vi "PipBoy_ConvertImageToIcon.vi"(8 "error in (no error)":errorcluster, 10 "Image":T1) -> (0 "error out":errorcluster, 2 "Icon":u16[][](array[numeric]))   [LabVIEW 2014]
uses:
  <vilib>/picture/picture.llb/imagedata.ctl
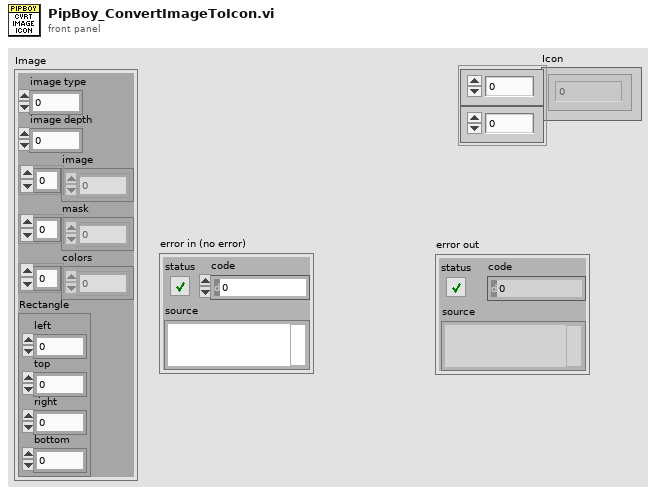
[diagram p1: front panel]
types:
  T1 = typedef "imagedata.ctl" = cluster{"image type":i32, "image depth":i32, "image":u8[], "mask":u8[], "colors":u32[], "Rectangle":cluster{"left":i16, "top":i16, "right":i16, "bottom":i16}}
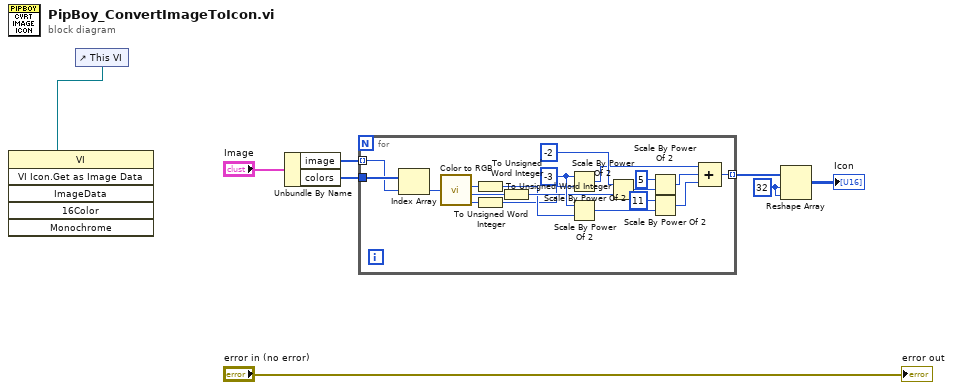
[diagram p0: block diagram]
diagram:
  w3 = 32 ("dimension size")
  n1 = control-ref of="This VI"() -> (w2:refnum<vi>)
  n2 = invoke class="VI" method="VI Icon.Get as Image Data"(reference=w2) -> ()  [unwired: 5 in, 6 out]
  n3 = Unbundle By Name("Image") -> ("image"=w6:u8[], "colors"=w5:u32[])
  n4 = for {
    tunnel: w6 -> [w26] mode=indexing
    tunnel: w5 -> [w27]
    tunnel: [w11] -> w4 mode=indexing
    w24 = i16 -3 ("n")
    n5 = Index Array(array=w27, index=w26) -> (element=w25:u32)
    n6 = call <vilib>:"Color to RGB.vi"("Color"=w25) -> ("R"=w20:u8, "G"=w19:u8, "B"=w17:u8)  [unwired: 1 out]
    n7 = To Unsigned Word Integer(number=w20) -> (unsigned 16bit integer=w10:u16)
    n8 = To Unsigned Word Integer(number=w17) -> (unsigned 16bit integer=w9:u16)
    n9 = To Unsigned Word Integer(number=w19) -> (unsigned 16bit integer=w18:u16)
    n10 = Scale By Power Of 2(n=w24, x=w9) -> (x*2^n=w14:u16)
    n11 = Scale By Power Of 2(n=w24, x=w10) -> (x*2^n=w16:u16)
    n12 = Scale By Power Of 2(n=i16 -2, x=w18) -> (x*2^n=w22:u16)
    n13 = Scale By Power Of 2(n=i16 5, x=w22) -> (x*2^n=w13:u16)
    n14 = Scale By Power Of 2(n=i16 11, x=w16) -> (x*2^n=w12:u16)
    n15 = Compound Arithmetic op=ADD(w14, w13, w12) -> (w11:u16)
  }
  n16 = Reshape Array(w4, w3, w3) -> (→"Icon":u16[][])
  "error out" <- "error in (no error)"
